vi "WinUtil Master.vi"(8 "error in (no error)":errorcluster, 10 "window enumeration info in":T1 {"process ID" format="%.0x"; "window handles" format="%.0x"}, 11 "function":T2(ring)) -> (0 "error out":errorcluster, 1 "window names":string[](array[string]), 2 "window enumeration info out":T1 {"process ID" format="%.0x"; "window handles" format="%.0x"})   [LabVIEW 2020, in "MacroAssert.lvlib" / "Winevent.lvlib"]
doc: "This VI has the ability to call three different functions in LVWUTIL.DLL. If called in succession, the Windows Task List can be programmatically generated. See Get Task List.vi. Calling these functions incorrectly can cause LabVIEW and / or Windows to crash!!"
uses:
  Winevent.lvlib
  LVWUtil32.dll
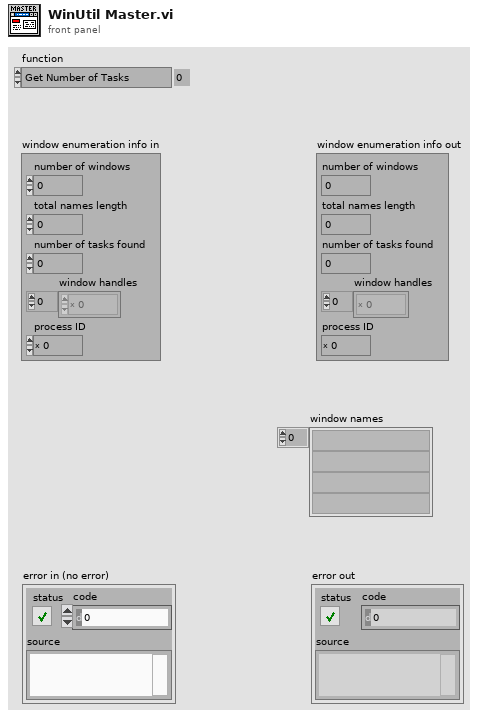
[diagram p1: front panel]
types:
  T1 = cluster{"number of windows":i32, "total names length":u32, "number of tasks found":i32, "window handles":u32[], "process ID":u32}
  T2 = enum16{"Get Number of Tasks", "Get Window Info", "Get Window Names"}
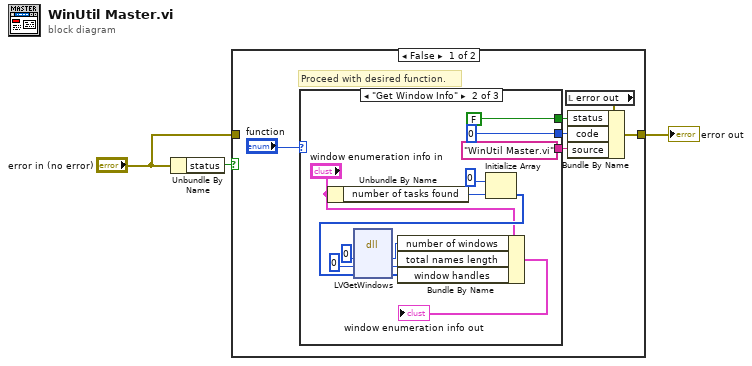
[diagram p0: block diagram]
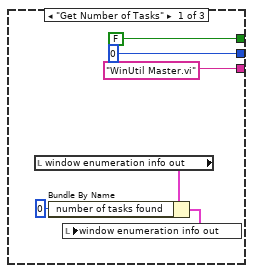
[diagram p2: hidden frame]
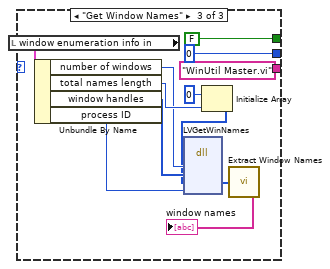
[diagram p3: hidden frame]
diagram:
  n1 = Unbundle By Name("error in (no error)") -> ("status"=w3:bool)
  n2 = case shown="False" w3 {
    tunnel: [w4 w41] -> w2
    tunnel: "error in (no error)" -> [_ w41]
    frame False {
      # "Proceed with desired function."
      n3 = case shown="\"Get Window Info\"" "function" {
        tunnel: [FALSE FALSE FALSE] -> w6
        tunnel: [0 0 0] -> w7
        tunnel: ["WinUtil Master.vi" "WinUtil Master.vi" "WinUtil Master.vi"] -> w8
        frame "Get Number of Tasks" {
          n4 = local read "window enumeration info out"() -> (w11:T1)
          n5 = Bundle By Name(cluster=w11, "number of tasks found"=0) -> (w10:T1)
          n6 = local write "window enumeration info out"(w10) -> ()
        }
        frame "Get Window Info" {
          n7 = Unbundle By Name("window enumeration info in") -> ("number of tasks found"=w24:i32)
          n8 = Initialize Array(u32 0, w24) -> (w21:u32[])
          n9 = dll-call lib="C:/Users/User/Documents/LabVIEW Data/Projects/MacroAssert/source/SubVIs/labview_win_util32_8.6/LVWUtil32.dll" fn="LVGetWindows"(0, u32 0, w21) -> (w18:i32, w19:u32, w20:u32[])  [unwired: 3 in, 3 out]
          n10 = Bundle By Name(cluster="window enumeration info in", "number of windows"=w18, "total names length"=w19, "window handles"=w20) -> (→"window enumeration info out":T1)
        }
        frame "Get Window Names" {
          n11 = local read "window enumeration info in"() -> (w36:T1)
          n12 = Unbundle By Name(w36) -> ("number of windows"=w34:i32, "total names length"=w35:u32, "window handles"=w33:u32[], "process ID"=w31:u32)
          n13 = Initialize Array(u8 0, w35) -> (w32:u8[])
          n14 = dll-call lib="C:/Users/User/Documents/LabVIEW Data/Projects/MacroAssert/source/SubVIs/labview_win_util32_8.6/LVWUtil32.dll" fn="LVGetWinNames"("numWin"=w34, w33, w32, "hInst"=w31) -> (w30:u8[])  [unwired: 6 in, 3 out]
          n15 = call "Extract Window Names.vi"("window names"=w30) -> ("application names"=→"window names":string[])
        }
      }
      n16 = local read "error out"() -> (w9:errorcluster)
      n17 = Bundle By Name(cluster=w9, "status"=w6, "code"=w7, "source"=w8) -> (w4:errorcluster)
    }
    frame True {
      # "Error has occured. Do not perform any window function."
    }
  }
  "error out" <- w2
